vi "Read OwnerTreeRefnum.vi"(8 "error in (no error)":errorcluster, 11 "Tag_LVOOP.lvclass in":refnum<class "Tree Tag Class.lvclass">) -> (0 "error out":errorcluster, 2 "Owner (Tree Refnum)":refnum<vi>, 3 "Tag_LVOOP.lvclass out":refnum<class "Tree Tag Class.lvclass">)   [LabVIEW 2012, in "Tree Tools.lvlib" / "Tree Tag Class.lvclass"]
uses:
  Tree Tag Class.lvclass
  Tree Tag Class.lvclass/Tree Tag Class.ctl
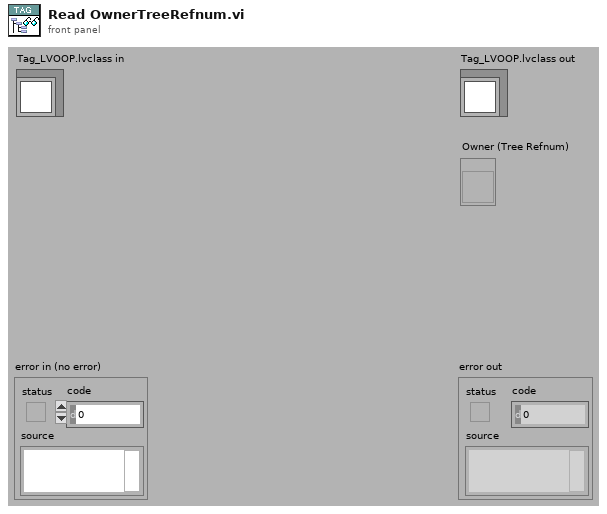
[diagram p1: front panel]
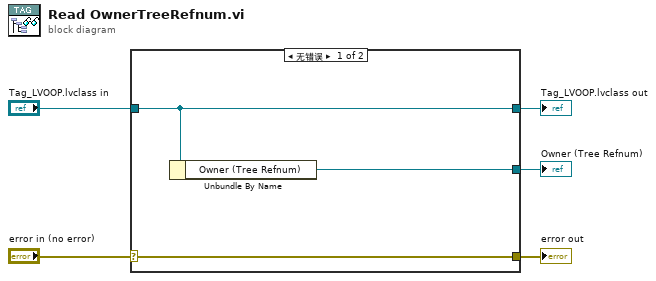
[diagram p0: block diagram]
diagram:
  n1 = case shown="无错误" "error in (no error)" {
    selector: "error in (no error)" -> [w8 w9]
    tunnel: [w8 w9] -> w4
    tunnel: [w7 w10] -> w2
    tunnel: "Tag_LVOOP.lvclass in" -> [w7 w10]
    tunnel: [w6 _] -> w1
    frame No Error {
      n2 = Unbundle By Name(w7) -> ("Owner (Tree Refnum)"=w6:refnum<vi>)
    }
    frame Error {
    }
  }
  "error out" <- w4
  "Tag_LVOOP.lvclass out" <- w2
  "Owner (Tree Refnum)" <- w1
